vi "RightClickMenu(Core).vi"(7 "datum":T1={"position"={"left"=200, "top"=200}, "font"={"name"="Tahoma", "size"=13, "color"=0}, "seperator color"=9868950, "frame color"=9868950, "overlay color"=26367}, 8 "error in (no error)":errorcluster, 11 "rcm file path":path=path "e:/_project/LabVIEW天下会/6th Round/LV Source/RCM File/NEW.xml") -> (0 "error out":errorcluster)   [LabVIEW 2009]
uses:
  <vilib>/Utility/miscctls.llb/LVPointTypeDef.ctl
  Class/Menu/menu.lvclass
panel:
  in  "queue name":string="RCM(Core)"
  in  "item name in":string
  out "menu":picture
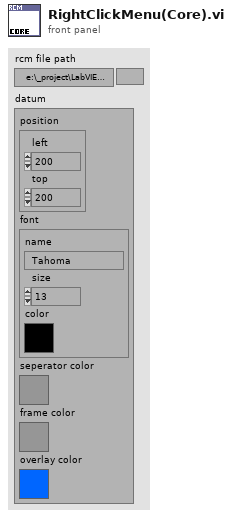
[diagram p1: front panel]
types:
  T1 = cluster{"position":cluster{"left":u32, "top":u32}, "font":cluster{"name":string, "size":i16, "color":u32}, "seperator color":u32, "frame color":u32, "overlay color":u32}
  T2 = typedef "LVPointTypeDef.ctl" = cluster{"Horizontal":i16, "Vertical":i16}
  T3 = typedef "RCMData.ctl" = cluster{"name":string, "icon path":path, "type":string, "parent?":bool}
  T4 = cluster{"left":i16, "top":i16, "right":i16, "bottom":i16}
  T5 = typedef "LVPoint32TypeDef.ctl" = cluster{"Horizontal":i32, "Vertical":i32}
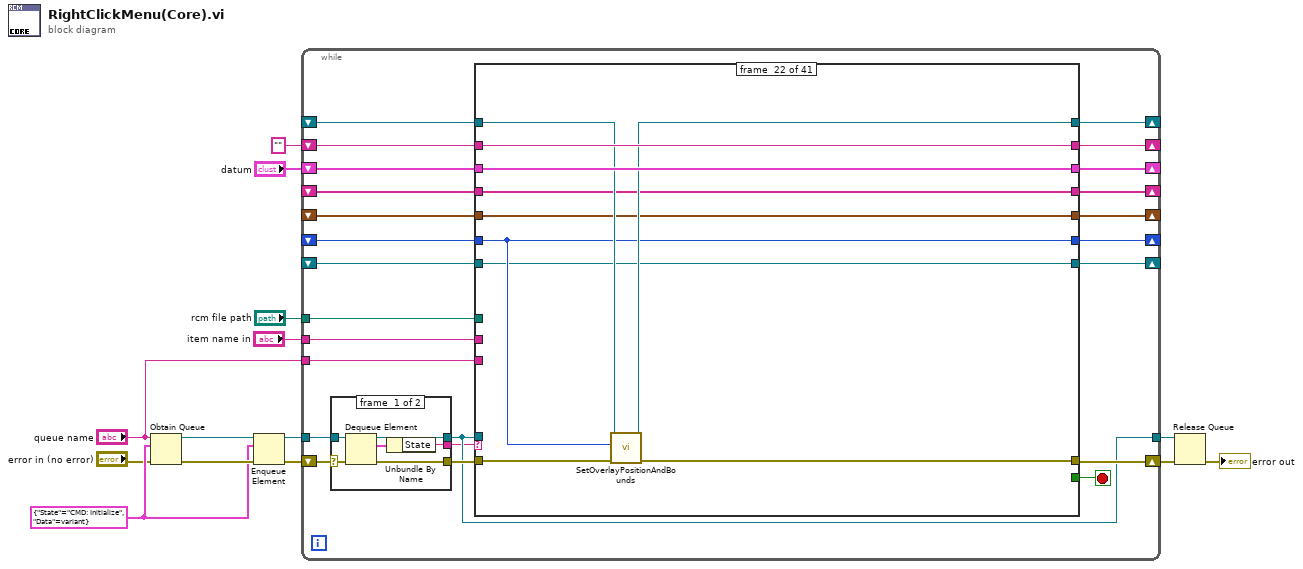
[diagram p0: block diagram]
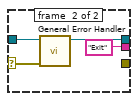
[diagram p2: hidden frame]
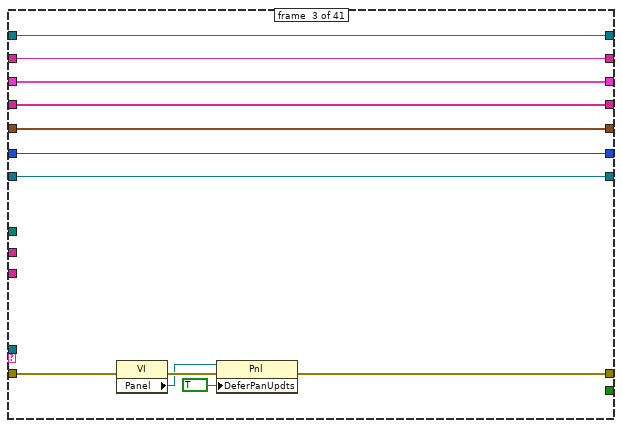
[diagram p5: hidden frame]
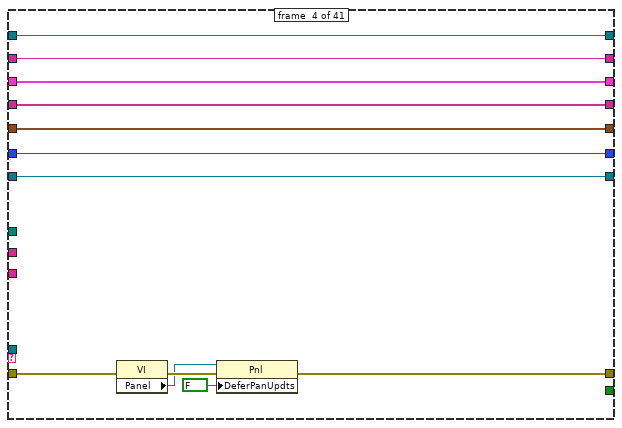
[diagram p6: hidden frame]
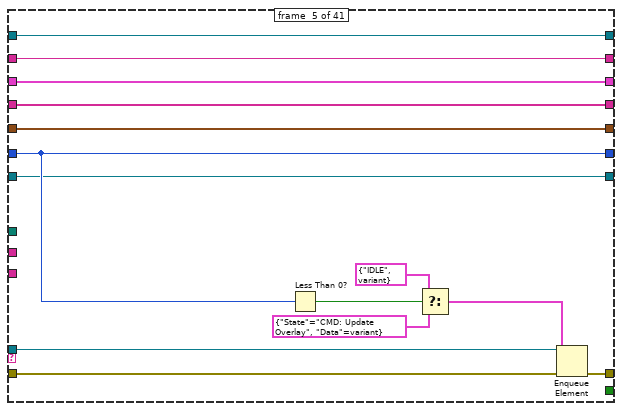
[diagram p7: hidden frame]
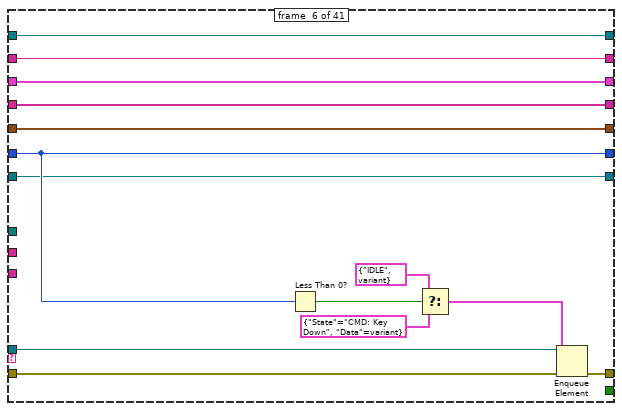
[diagram p8: hidden frame]
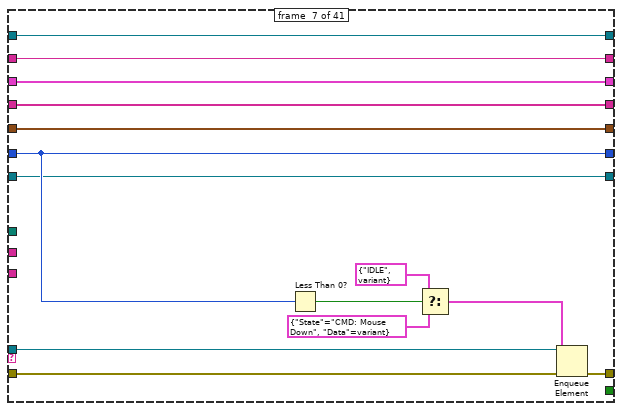
[diagram p9: hidden frame]
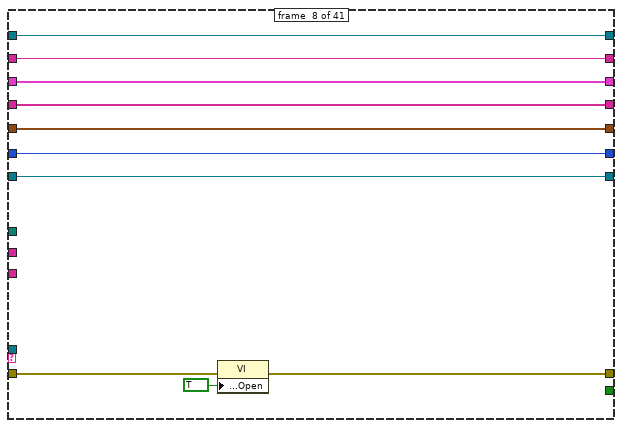
[diagram p10: hidden frame]
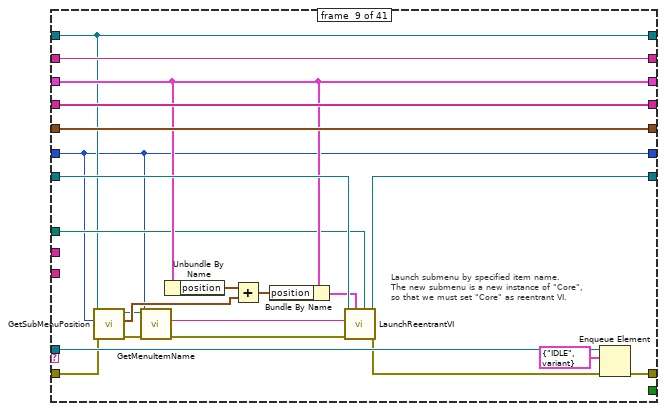
[diagram p11: hidden frame]
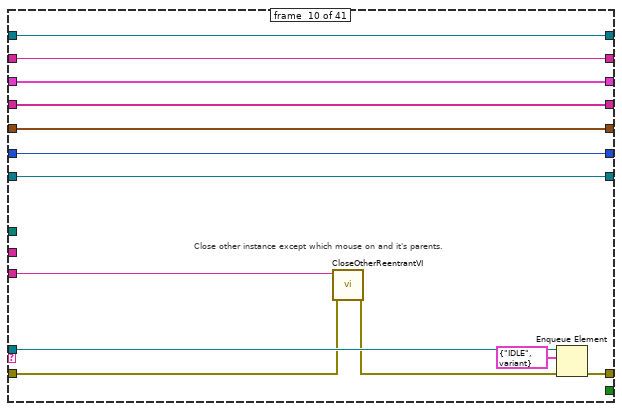
[diagram p12: hidden frame]
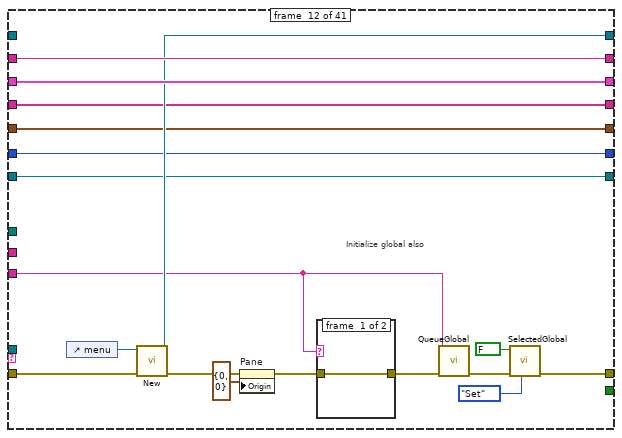
[diagram p14: hidden frame]
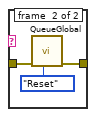
[diagram p15: hidden frame]
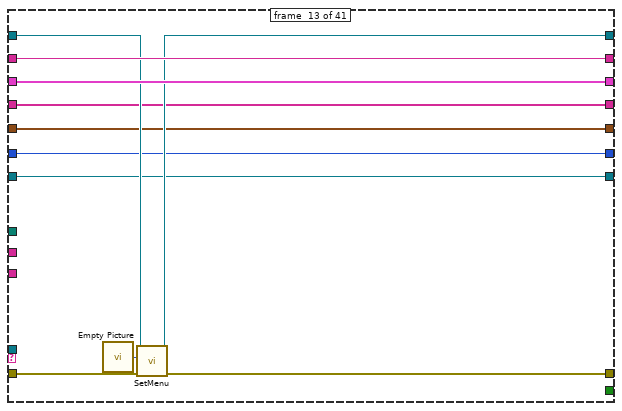
[diagram p16: hidden frame]
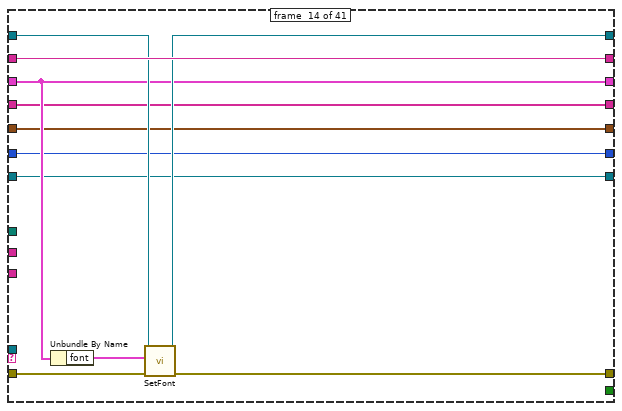
[diagram p17: hidden frame]
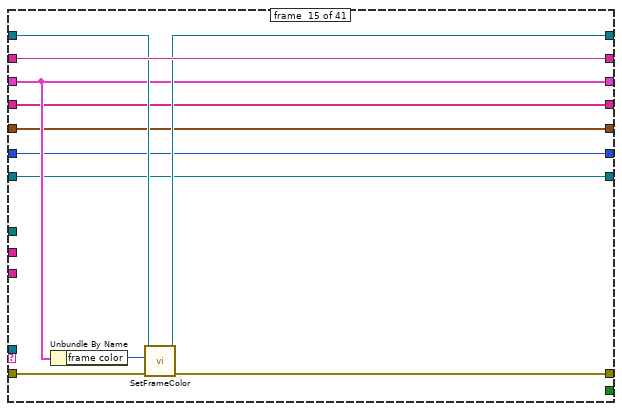
[diagram p18: hidden frame]
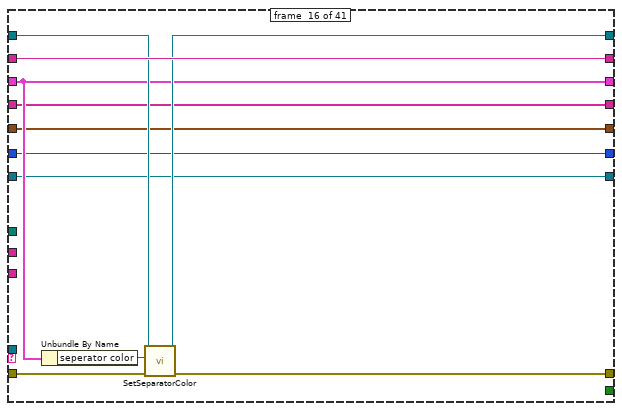
[diagram p19: hidden frame]
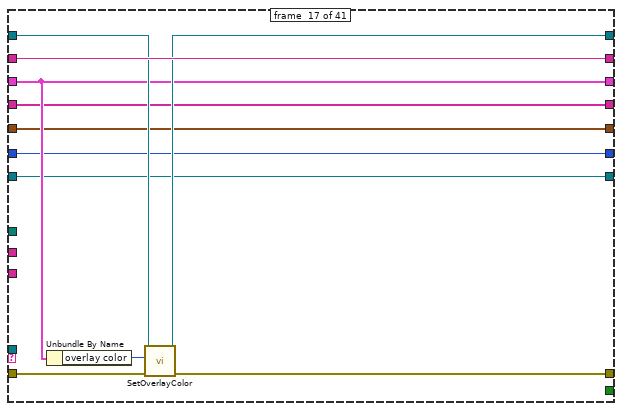
[diagram p20: hidden frame]
diagram:
  w9 = cluster{"State":string, "Data":variant} {"State"="CMD: Initialize", "Data"=variant}
  n1 = Obtain Queue(name (unnamed)="queue name", element data type=w9, error in (no error)="error in (no error)") -> (queue out=w6:refnum<queue>, error out=w14:errorcluster)  [unwired: 2 in, 1 out]
  n2 = Enqueue Element(queue=w6, element=w9, error in (no error)=w14) -> (queue out=w11:refnum<queue>, error out=w10:errorcluster)  [unwired: 2 out]
  n3 = while {
    tunnel: w11 -> [w37]
    shift-right: [w35] -> w12
    shift-left: w10 -> [w38]
    shift-right: [w33] -> _
    shift-left: _ -> [w34]
    shift-right: [w29] -> _
    shift-left: "" -> [w32]
    shift-right: [w30] -> _
    shift-left: "datum" -> [w31]
    tunnel: [w28] -> w13
    shift-right: [w25] -> _
    shift-left: _ -> [w24]
    shift-right: [w23] -> _
    shift-left: _ -> [w22]
    shift-right: [w21] -> _
    shift-left: _ -> [w20]
    shift-right: [w19] -> _
    shift-left: _ -> [w18]
    tunnel: "queue name" -> [w17]
    tunnel: "rcm file path" -> [w16]
    tunnel: "item name in" -> [w15]
    stop <- w27 stop-if-true
    n4 = case shown="No Error" w38 {
      selector: w38 -> [w43 w47]
      tunnel: w37 -> [w44 w46]
      tunnel: [w40 "Exit" ("State")] -> w26
      tunnel: [w42 _] -> w36
      tunnel: [w41 w46] -> w28
      frame #0 {
        n5 = Dequeue Element(queue=w44, error in (no error)=w43) -> (queue out=w41:refnum<queue>, element=w39:cluster{"State":string, "Data":variant}, error out=w42:errorcluster)  [unwired: 2 out]
        n6 = Unbundle By Name(w39) -> ("State"=w40:string)
      }
      frame #1 {
        n7 = call <vilib>:"General Error Handler.vi"("error in (no error)"=w47) -> ()  [unwired: 1 in, 14 out]
      }
    }
    n8 = case shown="\"----State----\"" w26 {
      tunnel: w36 -> [w55 w63 w75 w87 w91 w105 w119 w132 w153 w163 w182 w198 w213 w225 w236 w247 w258 w262 w281 w295 w305 w311 w322 w343 w352 w362 w372 w382 w390 w407 w427 w444 w522 w533 w548 w563 w578 w593 w608 w620 w622]
      tunnel: [w55 w63 w68 w80 w97 w111 w125 w131 w159 w171 w182 w185 w212 w224 w235 w246 w257 w274 w280 w294 w304 w312 w320 w338 w351 w361 w371 w381 w387 w409 w427 w443 w522 w529 w544 w559 w574 w589 w604 w620 w621] -> w35
      tunnel: w28 -> [_ _ _ _ w96 w110 w124 _ w158 w170 _ _ _ _ _ _ _ _ _ _ _ _ _ _ _ _ _ _ _ w406 _ w445 _ w528 w543 w558 w573 w588 w603 _ _]
      tunnel: w34 -> [w54 w62 w74 w86 w90 w104 w118 w135 w141 w169 w181 _ w210 w222 w233 w244 w255 w272 w283 w296 w306 w316 w325 w344 w353 w363 w373 w383 w401 w417 w426 w442 w521 w532 w547 w562 w577 w592 w607 w619 w630]
      tunnel: [w54 w62 w74 w86 w90 w104 w118 w135 w141 w169 w181 w195 w211 w223 w234 w245 w256 w273 w282 w293 w303 w315 w324 w341 w350 w360 w370 w380 w400 w416 w426 w441 w521 w532 w547 w562 w577 w592 w607 w619 w630] -> w33
      tunnel: w32 -> [w52 w60 w72 w84 w101 w115 w129 w139 w161 w174 w179 w199 w214 w226 w237 w248 w259 w275 w288 w298 w308 w318 w328 w345 w355 w365 w375 w385 w403 w419 w424 w440 w519 w530 w545 w560 w575 w590 w605 w617 w628]
      tunnel: w31 -> [w53 w61 w73 w85 w100 w114 w128 w138 w149 w166 w180 w200 w215 w221 w232 w243 w254 w271 w287 w297 w307 w317 w327 w337 w354 w364 w374 w384 w402 w418 w425 w439 w520 w531 w546 w561 w576 w591 w606 w618 w629]
      tunnel: [w53 w61 w73 w85 w100 w114 w128 w138 w149 w166 w180 w200 w215 w221 w232 w243 w254 w271 w287 w297 w307 w317 w327 w337 w354 w364 w374 w384 w402 w418 w425 w438 w520 w531 w546 w561 w576 w591 w606 w618 w629] -> w30
      tunnel: [w52 w60 w72 w84 w101 w115 w129 w139 w161 w174 w179 w199 w214 w226 w237 w248 w259 w275 w288 w298 w308 w318 w328 w345 w355 w365 w375 w385 w403 w419 w424 w437 w519 w530 w545 w560 w575 w590 w605 w617 w628] -> w29
      tunnel: [_ _ _ _ _ _ _ _ _ _ _ _ _ _ _ _ _ _ _ _ _ _ _ _ _ _ _ _ _ _ _ _ _ _ _ _ _ _ _ _ TRUE] -> w27
      tunnel: [w51 w59 w71 w83 w99 w113 w127 w137 w160 w173 w178 w194 w208 w219 w230 w241 w252 w270 w279 w292 w302 w314 w326 w342 w349 w359 w369 w379 w397 w413 w423 w435 w518 w526 w541 w556 w571 w586 w601 w616 w626] -> w25
      tunnel: w24 -> [w51 w59 w71 w83 w99 w113 w127 w137 w160 w173 w178 w194 w208 w219 w230 w241 w252 w270 w279 w292 w302 w314 w326 w342 w349 w359 w369 _ w397 w413 w423 w436 w518 w526 w541 w556 w571 w586 w601 w616 w626]
      tunnel: [w50 w58 w66 w78 w98 w112 w126 w136 w150 w172 w177 w192 w207 w218 w229 w240 w251 w269 w278 w291 w301 w313 w323 w333 w348 w358 w368 w378 w399 w415 w422 w434 w517 w525 w540 w555 w570 w585 w600 w615 w625] -> w23
      tunnel: w22 -> [w50 w58 w66 w78 w98 w112 w126 w136 w150 w172 w177 w192 w207 w218 w229 w240 w251 w269 w278 w291 w301 w313 w323 w333 w348 w358 w368 w378 w399 w415 w422 w433 w517 w525 w540 w555 w570 w585 w600 w615 w625]
      tunnel: [w49 w57 w65 w77 w89 w103 w117 w134 w140 w168 w176 w191 w206 w217 w228 w239 w250 w268 w277 w290 w300 w310 w321 w332 w347 w357 w367 w377 w398 w414 w421 w431 w516 w524 w539 w554 w569 w584 w599 w614 w624] -> w21
      tunnel: w20 -> [w49 w57 w65 w77 w89 w103 w117 w134 w140 w168 w176 w191 w206 w217 w228 w239 w250 w268 w277 w290 w300 w310 _ w332 w347 w357 w367 w377 w398 w414 w421 w432 w516 w524 w539 w554 w569 w584 w599 w614 w624]
      tunnel: [w48 w56 w64 w76 w88 w102 w116 w133 w154 w164 w175 w190 w205 w216 w227 w238 w249 w267 w276 w289 w299 w309 w319 w330 w346 w356 w366 w376 w396 w404 w420 w429 w515 w523 w538 w553 w568 w583 w598 w613 w623] -> w19
      tunnel: w18 -> [w48 w56 w64 w76 w88 w102 w116 w133 w155 w164 w175 w190 w205 w216 w227 w238 w249 w267 w276 w289 w299 w309 w319 w330 w346 w356 w366 w376 w396 w404 w420 w430 w515 w523 w538 w553 w568 w583 w598 w613 w623]
      tunnel: w17 -> [_ _ _ _ _ _ _ _ _ w165 _ w186 _ _ _ _ _ _ _ _ _ _ _ _ _ _ _ _ w395 _ _ _ _ _ _ _ _ _ _ _ _]
      tunnel: w16 -> [_ _ _ _ _ _ _ _ w147 _ _ _ _ _ _ _ _ w266 _ _ _ _ _ _ _ _ _ _ _ _ _ _ _ _ _ _ _ _ _ _ _]
      tunnel: w15 -> [_ _ _ _ _ _ _ _ _ _ _ _ _ _ _ _ _ w265 _ _ _ _ _ _ _ _ _ _ _ _ _ _ _ _ _ _ _ _ _ _ _]
      frame #0 {
      }
      frame #1 {
      }
      frame #2 {
        n9 = property class="VI"(error in=w75) -> (error out=w70:errorcluster, "Panel"=w69:refnum<vi>)  [unwired: 1 in, 1 out]
        n10 = property class="Pnl"(reference=w69, error in=w70, "DeferPanUpdts"=TRUE ("Defer Panel Updates")) -> (error out=w68:errorcluster)  [unwired: 1 out]
      }
      frame #3 {
        n11 = property class="VI"(error in=w87) -> (error out=w82:errorcluster, "Panel"=w81:refnum<vi>)  [unwired: 1 in, 1 out]
        n12 = property class="Pnl"(reference=w81, error in=w82, "DeferPanUpdts"=FALSE ("Defer Panel Updates")) -> (error out=w80:errorcluster)  [unwired: 1 out]
      }
      frame #4 {
        n13 = Less Than 0?(x=w89) -> (x < 0?=w93:bool)
        n14 = Select(t=cluster{"State":string, "Data":variant} {"State"="IDLE", "Data"=variant} ("element"), s=w93, f=cluster{"State":string, "Data":variant} {"State"="CMD: Update Overlay", "Data"=variant} ("element")) -> (s? t:f=w92:cluster{"State":string, "Data":variant})
        n15 = Enqueue Element(queue=w96, element=w92, error in (no error)=w91) -> (error out=w97:errorcluster)  [unwired: 1 in, 2 out]
      }
      frame #5 {
        n16 = Less Than 0?(x=w103) -> (x < 0?=w107:bool)
        n17 = Select(t=cluster{"State":string, "Data":variant} {"State"="IDLE", "Data"=variant} ("element"), s=w107, f=cluster{"State":string, "Data":variant} {"State"="CMD: Key Down", "Data"=variant} ("element")) -> (s? t:f=w106:cluster{"State":string, "Data":variant})
        n18 = Enqueue Element(queue=w110, element=w106, error in (no error)=w105) -> (error out=w111:errorcluster)  [unwired: 1 in, 2 out]
      }
      frame #6 {
        n19 = Less Than 0?(x=w117) -> (x < 0?=w121:bool)
        n20 = Select(t=cluster{"State":string, "Data":variant} {"State"="IDLE", "Data"=variant} ("element"), s=w121, f=cluster{"State":string, "Data":variant} {"State"="CMD: Mouse Down", "Data"=variant} ("element")) -> (s? t:f=w120:cluster{"State":string, "Data":variant})
        n21 = Enqueue Element(queue=w124, element=w120, error in (no error)=w119) -> (error out=w125:errorcluster)  [unwired: 1 in, 2 out]
      }
      frame #7 {
        n22 = property class="VI"(error in=w132, "Front Panel.Open"=TRUE ("Front Panel Window:Open")) -> (error out=w131:errorcluster)  [unwired: 1 in, 1 out]
      }
      frame #8 {
        # "Launch submenu by specified item name.\nThe new submenu is a new instance of \"Core\",\nso that we must set \"Core\" as reentrant VI."
        n23 = call "GetSubMenuPosition.vi"("error in (no error)"=w153, "index"=w140, "menu in"=w141) -> ("error out"=w145:errorcluster, "position"=w151:cluster{"left":u32, "top":u32}, "menu out"=w143:refnum<class "menu.lvclass">)  [unwired: 6 in]
        n24 = call "GetMenuItemName.vi"("error in (no error)"=w145, "menu item index"=w140, "menu in"=w143) -> ("error out"=w144:errorcluster, "item name"=w142:string)  [unwired: 6 in, 1 out]
        n25 = Unbundle By Name(w149) -> ("position"=w148:cluster{"left":u32, "top":u32})
        n26 = Add(x=w148, y=w151) -> (x+y=w152:cluster{"left":u32, "top":u32})
        n27 = Bundle By Name(cluster=w149, "position"=w152) -> (w146:T1)
        n28 = call "LaunchReentrantVI.vi"("rcm file path"=w147, "datum"=w146, "error in (no error)"=w144, "item name in"=w142, "vi reference in"=w155) -> ("error out"=w156:errorcluster, "vi reference out"=w154:refnum<vi>)  [unwired: 5 in]
        n29 = Enqueue Element(queue=w158, element=cluster{"State":string, "Data":variant} {"State"="IDLE", "Data"=variant}, error in (no error)=w156) -> (error out=w159:errorcluster)  [unwired: 1 in, 2 out]
      }
      frame #9 {
        # "Close other instance except which mouse on and it's parents."
        n30 = call "CloseOtherReentrantVI.vi"("error in (no error)"=w163, "current queue name"=w165) -> ("error out"=w162:errorcluster)  [unwired: 9 in]
        n31 = Enqueue Element(queue=w170, element=cluster{"State":string, "Data":variant} {"State"="IDLE", "Data"=variant}, error in (no error)=w162) -> (error out=w171:errorcluster)  [unwired: 1 in, 2 out]
      }
      frame #10 {
      }
      frame #11 {
        # "Initialize global also"
        n32 = control-ref of="menu"() -> (w196:refnum<vi>)
        n33 = call "New.vi"("error in (no error)"=w198, "menu refnum"=w196) -> ("error out"=w197:errorcluster, "menu out"=w195:refnum<class "menu.lvclass">)  [unwired: 8 in]
        n34 = property on="Pane" class="Pane"(error in=w197, "Origin"=T2 {"Horizontal"=0, "Vertical"=0}) -> (error out=w188:errorcluster)  [unwired: 1 in, 1 out]
        n35 = case shown="\"RCM(Core)\"" w186 {
          tunnel: w188 -> [w201 w203]
          tunnel: [w201 w202] -> w187
          frame #0 {
          }
          frame #1 {
            n36 = call "QueueGlobal.vi"("cmd (Add)"=enum16{"Add One to End", "Get All", "Reset"}."Reset", "error in (no error)"=w203) -> ("error out"=w202:errorcluster)  [unwired: 8 in, 1 out]
          }
        }
        n37 = call "QueueGlobal.vi"("error in (no error)"=w187, "queue name"=w186) -> ("error out"=w189:errorcluster)  [unwired: 8 in, 1 out]
        n38 = call "SelectedGlobal.vi"("cmd(Get)"=enum16{"Get", "Set"}."Set", "error in (no error)"=w189, "selected in"=FALSE ("cancel")) -> ("error out"=w185:errorcluster)  [unwired: 7 in, 1 out]
      }
      frame #12 {
        n39 = call "Empty Picture"() -> ("empty picture"=w209:picture)
        n40 = call "SetMenu.vi"("error in (no error)"=w213, "menu"=w209, "menu in"=w210) -> ("error out"=w212:errorcluster, "menu out"=w211:refnum<class "menu.lvclass">)  [unwired: 7 in]
      }
      frame #13 {
        n41 = Unbundle By Name(w221) -> ("font"=w220:cluster{"name":string, "size":i16, "color":u32})
        n42 = call "SetFont.vi"("error in (no error)"=w225, "font"=w220, "menu in"=w222) -> ("error out"=w224:errorcluster, "menu out"=w223:refnum<class "menu.lvclass">)  [unwired: 7 in]
      }
      frame #14 {
        n43 = Unbundle By Name(w232) -> ("frame color"=w231:u32)
        n44 = call "SetFrameColor.vi"("error in (no error)"=w236, "frame color"=w231, "menu in"=w233) -> ("error out"=w235:errorcluster, "menu out"=w234:refnum<class "menu.lvclass">)  [unwired: 7 in]
      }
      frame #15 {
        n45 = Unbundle By Name(w243) -> ("seperator color"=w242:u32)
        n46 = call "SetSeparatorColor.vi"("error in (no error)"=w247, "separator color"=w242, "menu in"=w244) -> ("error out"=w246:errorcluster, "menu out"=w245:refnum<class "menu.lvclass">)  [unwired: 7 in]
      }
      frame #16 {
        n47 = Unbundle By Name(w254) -> ("overlay color"=w253:u32)
        n48 = call "SetOverlayColor.vi"("error in (no error)"=w258, "overlay color"=w253, "menu in"=w255) -> ("error out"=w257:errorcluster, "menu out"=w256:refnum<class "menu.lvclass">)  [unwired: 7 in]
      }
      frame #17 {
        # "Use dynamic dispaching to generate menu item objects array"
        n49 = call "ReadRCMFileToRCMDatum.vi"("error in (no error)"=w262, "item name (\"\": root)"=w265, "rcm file path"=w266) -> ("error out"=w263:errorcluster, "rcm datum"=w264:T3[])  [unwired: 7 in]
        n50 = call "RCMDatumToMenuItems.vi"("error in (no error)"=w263, "rcm datum"=w264) -> ("error out"=w261:errorcluster, "menu items"=w260:refnum<class "menu item.lvclass">[])  [unwired: 8 in]
        n51 = call "SetMenuItems.vi"("error in (no error)"=w261, "menu items"=w260, "menu in"=w272) -> ("error out"=w274:errorcluster, "menu out"=w273:refnum<class "menu.lvclass">)  [unwired: 7 in]
      }
      frame #18 {
        n52 = call "CalculateBounds.vi"("error in (no error)"=w281, "menu in"=w283) -> ("error out"=w285:errorcluster, "bounds"=w284:cluster{"width":u32, "height":u32}, "menu out"=w286:refnum<class "menu.lvclass">)  [unwired: 7 in]
        n53 = call "SetBounds.vi"("error in (no error)"=w285, "bounds"=w284, "menu in"=w286) -> ("error out"=w280:errorcluster, "menu out"=w282:refnum<class "menu.lvclass">)  [unwired: 7 in]
      }
      frame #19 {
        n54 = call "SetFrameBounds.vi"("error in (no error)"=w295, "menu in"=w296) -> ("error out"=w294:errorcluster, "menu out"=w293:refnum<class "menu.lvclass">)  [unwired: 8 in]
      }
      frame #20 {
        n55 = call "SetMenuItemsPositionAndBounds.vi"("error in (no error)"=w305, "menu in"=w306) -> ("error out"=w304:errorcluster, "menu out"=w303:refnum<class "menu.lvclass">)  [unwired: 8 in]
      }
      frame #21 {
        n56 = call "SetOverlayPositionAndBounds.vi"("error in (no error)"=w311, "item index"=w310, "menu in"=w316) -> ("error out"=w312:errorcluster, "menu out"=w315:refnum<class "menu.lvclass">)  [unwired: 7 in]
      }
      frame #22 {
        n57 = call "CalculateMenuItemIndex.vi"("error in (no error)"=w322, "position"=w323, "menu in"=w325) -> ("error out"=w320:errorcluster, "menu item index"=w321:i32, "menu out"=w324:refnum<class "menu.lvclass">)  [unwired: 6 in]
      }
      frame #23 {
        # "Set menu size"
        n58 = Unbundle By Name(w337) -> ("position"=w334:cluster{"left":u32, "top":u32})
        n59 = call "SetDrawAreaSize.vi"("error in (no error)"=w343, "menu in"=w344) -> ("error out"=w340:errorcluster, "menu out"=w341:refnum<class "menu.lvclass">)  [unwired: 8 in]
        n60 = call "GetBounds.vi"("error in (no error)"=w340, "menu in"=w341) -> ("error out"=w339:errorcluster, "bounds"=w336:cluster{"width":u32, "height":u32})  [unwired: 7 in, 1 out]
        n61 = Add(x=w334, y=w336) -> (x+y=w335:cluster{u32, u32})
        n62 = call <vilib>:"Point2Rect.vi"("point b"=w335, "point a"=w334) -> ("rect"=w331:T4)
        n63 = control-ref of="This VI"() -> (w329:refnum<vi>)
        n64 = property class="VI"(reference=w329, error in=w339, "Front Panel.PanelBounds"=w331) -> (error out=w338:errorcluster)  [unwired: 1 out]
      }
      frame #24 {
        n65 = call "DrawFrame.vi"("error in (no error)"=w352, "menu in"=w353) -> ("error out"=w351:errorcluster, "menu out"=w350:refnum<class "menu.lvclass">)  [unwired: 8 in]
      }
      frame #25 {
        n66 = call "DrawOverlay.vi"("error in (no error)"=w362, "menu in"=w363) -> ("error out"=w361:errorcluster, "menu out"=w360:refnum<class "menu.lvclass">)  [unwired: 8 in]
      }
      frame #26 {
        # "Use factory pattern to draw menu items dynamically"
        n67 = call "DrawMenuItems.vi"("error in (no error)"=w372, "menu in"=w373) -> ("error out"=w371:errorcluster, "menu out"=w370:refnum<class "menu.lvclass">)  [unwired: 8 in]
      }
      frame #27 {
        n68 = call "GetShortcuts.vi"("error in (no error)"=w382, "menu in"=w383) -> ("error out"=w381:errorcluster, "shortcuts"=w379:string[], "menu out"=w380:refnum<class "menu.lvclass">)  [unwired: 7 in]
      }
      frame #28 {
        n69 = call "ExitAllReentrantVI.vi"("error in (no error)"=w390, "current queue name"=w395) -> ("error out"=w391:errorcluster)  [unwired: 9 in]
        n70 = call "GetMenuItemName.vi"("error in (no error)"=w391, "menu item index"=w398, "menu in"=w401) -> ("error out"=w393:errorcluster, "item name"=w394:string, "menu out"=w400:refnum<class "menu.lvclass">)  [unwired: 6 in]
        n71 = call "ItemNameGlobal.vi"("cmd(Get)"=enum16{"Get", "Set"}."Set", "error in (no error)"=w393, "item name in"=w394) -> ("error out"=w388:errorcluster)  [unwired: 7 in, 1 out]
        n72 = call "SelectedGlobal.vi"("cmd(Get)"=enum16{"Get", "Set"}."Set", "error in (no error)"=w388, "selected in"=TRUE ("cancel")) -> ("error out"=w387:errorcluster)  [unwired: 7 in, 1 out]
      }
      frame #29 {
        # "Launch new submenu when it's parent."
        n73 = call "IsParent.vi"("error in (no error)"=w407, "index"=w414, "menu in"=w417) -> ("error out"=w408:errorcluster, "parent?"=w405:bool, "menu out"=w416:refnum<class "menu.lvclass">)  [unwired: 6 in]
        n74 = Select(t=cluster{"State":string, "Data":variant} {"State"="State: Launch", "Data"=variant} ("element"), s=w405, f=cluster{"State":string, "Data":variant} {"State"="State: Dispose", "Data"=variant} ("element")) -> (s? t:f=w410:cluster{"State":string, "Data":variant})
        n75 = Enqueue Element(queue=w406, element=w410, error in (no error)=w408) -> (error out=w409:errorcluster)  [unwired: 1 in, 2 out]
      }
      frame #30 {
      }
      frame #31 {
        n76 = event shown="[0] Panel Close?" {
          selector: _ -> [_ _ _ _ _]
          dyn-events: _ -> [_ _ _ _ _]
          timeout: 10 -> [_ _ _ _ _]
          tunnel: w445 -> [w452 w463 w474 w485 w504]
          tunnel: w444 -> [w453 w464 w475 w486 w505]
          tunnel: [w457 w468 w479 w490 w509] -> w443
          tunnel: w442 -> [w456 w467 w478 w489 w508]
          tunnel: [w456 w467 w478 w489 w508] -> w441
          tunnel: w440 -> [w455 w466 w477 w488 w507]
          tunnel: w439 -> [w454 w465 w476 w487 w506]
          tunnel: [w454 w465 w476 w487 w506] -> w438
          tunnel: [w455 w466 w477 w488 w507] -> w437
          tunnel: w436 -> [w449 w461 w473 w484 w500]
          tunnel: [w449 w461 w473 w484 w500] -> w435
          tunnel: [w448 w460 w471 w482 w502] -> w434
          tunnel: w433 -> [w448 w460 _ _ w502]
          tunnel: w432 -> [w447 w459 w470 w481 _]
          tunnel: [w447 w459 w470 w481 w492] -> w431
          tunnel: w430 -> [w446 w458 w469 w480 w495]
          tunnel: [w446 w458 w469 w480 w495] -> w429
          event #0 {
            n77 = event-data() -> ()  [unwired: 2 out]
            n78 = event-data("Discard?"=TRUE) -> ()  [unwired: 1 in, 1 out]
            n79 = Enqueue Element(queue=w452, element=cluster{"State":string, "Data":variant} {"State"="Exit", "Data"=variant}, error in (no error)=w453) -> (error out=w457:errorcluster)  [unwired: 3 out]
          }
          event #1 {
            n80 = event-data() -> ()  [unwired: 2 out]
            n81 = Enqueue Element(queue=w463, element=cluster{"State":string, "Data":variant} {"State"="IDLE", "Data"=variant}, error in (no error)=w464) -> (error out=w468:errorcluster)  [unwired: 3 out]
          }
          event #2 {
            n82 = event-data() -> ("Coords"=w471:T5)  [unwired: 1 out]
            n83 = Enqueue Element(queue=w474, element=cluster{"State":string, "Data":variant} {"State"="CMD: Overlay Check", "Data"=variant}, error in (no error)=w475) -> (error out=w479:errorcluster)  [unwired: 3 out]
          }
          event #3 {
            n84 = event-data() -> ("Coords"=w482:T5)  [unwired: 1 out]
            n85 = Enqueue Element(queue=w485, element=cluster{"State":string, "Data":variant} {"State"="CMD: Mouse Down Check", "Data"=variant}, error in (no error)=w486) -> (error out=w490:errorcluster)  [unwired: 3 out]
          }
          event #4 {
            n86 = event-data() -> ("Char"=w501:i16)  [unwired: 1 out]
            n87 = To Unsigned Byte Integer(number=w501) -> (unsigned 8bit integer=w498:u8)
            n88 = Type Cast(x=w498) -> (*(type *) &x=w499:string)  [unwired: 1 in]
            n89 = To Lower Case(string=w500) -> (all lower case string=w497:string[])
            n90 = To Lower Case(string=w499) -> (all lower case string=w496:string)
            n91 = for "Check shortcut" {
              tunnel: [w513] -> w493
              tunnel: w497 -> [w512] mode=indexing
              tunnel: w496 -> [w511]
              tunnel: [w510] -> w494
              i -> [w513]
              stop <- w510 stop-if-true
              n92 = Match Pattern(string=w512, regular expression=w511) -> (offset past match=w514:i32)  [unwired: 1 in, 3 out]
              n93 = Greater Or Equal To 0?(x=w514) -> (x >= 0?=w510:bool)
            }
            n94 = Select(t=w493, s=w494, f=-1) -> (s? t:f=w492:i32)
            n95 = Enqueue Element(queue=w504, element=cluster{"State":string, "Data":variant} {"State"="State: Right Key Down?", "Data"=variant}, error in (no error)=w505) -> (error out=w509:errorcluster)  [unwired: 3 out]
          }
        }
      }
      frame #32 {
      }
      frame #33 {
        n96 = for {
          tunnel: w528 -> [w535]
          shift-right: [w536] -> w529
          shift-left: w533 -> [w537]
          tunnel: cluster{"State":string, "Data":variant}[] [{"State"="Menu: New", "Data"=variant}, {"State"="Menu: Empty", "Data"=variant}, {"State"="Menu: Set Font", "Data"=variant}, {"State"="Menu: Set Frame Color", "Data"=variant}, {"State"="Menu: Set Overlay Color", "Data"=variant}, {"State"="Menu: Set Seperator Color", "Data"=variant}, {"State"="Menu: Set Menu Items", "Data"=variant}, {"State"="Menu: Set Bounds", "Data"=variant}, {"State"="Menu: Set Frame Bounds", "Data"=variant}, {"State"="Menu: Set Menu Items Position and Bounds", "Data"=variant}, {"State"="Menu: Draw Frame", "Data"=variant}, {"State"="Menu: Draw Menu Items", "Data"=variant}, {"State"="Menu: Get Shortcuts", "Data"=variant}, {"State"="Menu: Set Draw Area Size", "Data"=variant}, {"State"="State: Open FP", "Data"=variant}, {"State"="IDLE", "Data"=variant}] -> [w534] mode=indexing
          n97 = Enqueue Element(queue=w535, element=w534, error in (no error)=w537) -> (error out=w536:errorcluster)  [unwired: 1 in, 2 out]
        }
      }
      frame #34 {
        n98 = for {
          tunnel: w543 -> [w550]
          shift-right: [w551] -> w544
          shift-left: w548 -> [w552]
          tunnel: cluster{"State":string, "Data":variant}[] [{"State"="Menu: Calculate Menu Item Index", "Data"=variant}, {"State"="State: Update Overlay?", "Data"=variant}] -> [w549] mode=indexing
          n99 = Enqueue Element(queue=w550, element=w549, error in (no error)=w552) -> (error out=w551:errorcluster)  [unwired: 1 in, 2 out]
        }
      }
      frame #35 {
        n100 = for {
          tunnel: w558 -> [w565]
          shift-right: [w566] -> w559
          shift-left: w563 -> [w567]
          tunnel: cluster{"State":string, "Data":variant}[] [{"State"="Menu: Set Overlay Position and Bounds", "Data"=variant}, {"State"="State: Defer Update", "Data"=variant}, {"State"="Menu: Empty", "Data"=variant}, {"State"="Menu: Draw Frame", "Data"=variant}, {"State"="Menu: Draw Overlay", "Data"=variant}, {"State"="Menu: Draw Menu Items", "Data"=variant}, {"State"="State: Allow Update", "Data"=variant}, {"State"="Menu: Is Parent?", "Data"=variant}] -> [w564] mode=indexing
          n101 = Enqueue Element(queue=w565, element=w564, error in (no error)=w567) -> (error out=w566:errorcluster)  [unwired: 1 in, 2 out]
        }
      }
      frame #36 {
        n102 = for {
          tunnel: w573 -> [w580]
          shift-right: [w581] -> w574
          shift-left: w578 -> [w582]
          tunnel: cluster{"State":string, "Data":variant}[] [{"State"="Menu: Get Menu Item Name", "Data"=variant}, {"State"="Exit", "Data"=variant}] -> [w579] mode=indexing
          n103 = Enqueue Element(queue=w580, element=w579, error in (no error)=w582) -> (error out=w581:errorcluster)  [unwired: 1 in, 2 out]
        }
      }
      frame #37 {
        n104 = for {
          tunnel: w588 -> [w595]
          shift-right: [w596] -> w589
          shift-left: w593 -> [w597]
          tunnel: cluster{"State":string, "Data":variant}[] [{"State"="Menu: Calculate Menu Item Index", "Data"=variant}, {"State"="State: Right Mouse Down?", "Data"=variant}] -> [w594] mode=indexing
          n105 = Enqueue Element(queue=w595, element=w594, error in (no error)=w597) -> (error out=w596:errorcluster)  [unwired: 1 in, 2 out]
        }
      }
      frame #38 {
        n106 = for {
          tunnel: w603 -> [w610]
          shift-right: [w611] -> w604
          shift-left: w608 -> [w612]
          tunnel: cluster{"State":string, "Data":variant}[] [{"State"="Menu: Get Menu Item Name", "Data"=variant}, {"State"="Exit", "Data"=variant}] -> [w609] mode=indexing
          n107 = Enqueue Element(queue=w610, element=w609, error in (no error)=w612) -> (error out=w611:errorcluster)  [unwired: 1 in, 2 out]
        }
      }
      frame #39 {
      }
      frame #40 {
        n108 = invoke class="VI" method="FP.Close"(error in=w622) -> (error out=w621:errorcluster)  [unwired: 2 in, 2 out]
      }
    }
  }
  n109 = Release Queue(queue=w13, error in (no error)=w12) -> (error out=→"error out":errorcluster)  [unwired: 3 out]
